vi "requireDataFromPort.vi"(3 "error in (no error)":errorcluster, 4 "Command":string, 5 "VISA resource name":refnum<visa-resource-name>="COM1" caption="端口号") -> (0 "error out":errorcluster, 1 "Data":string, 2 "VISA resource name 2":refnum<visa-resource-name>="COM1" caption="端口号")   [LabVIEW 2010]
panel:
  out "波形图表":dbl(graph)
  out "数值":dbl
  out "布尔":bool
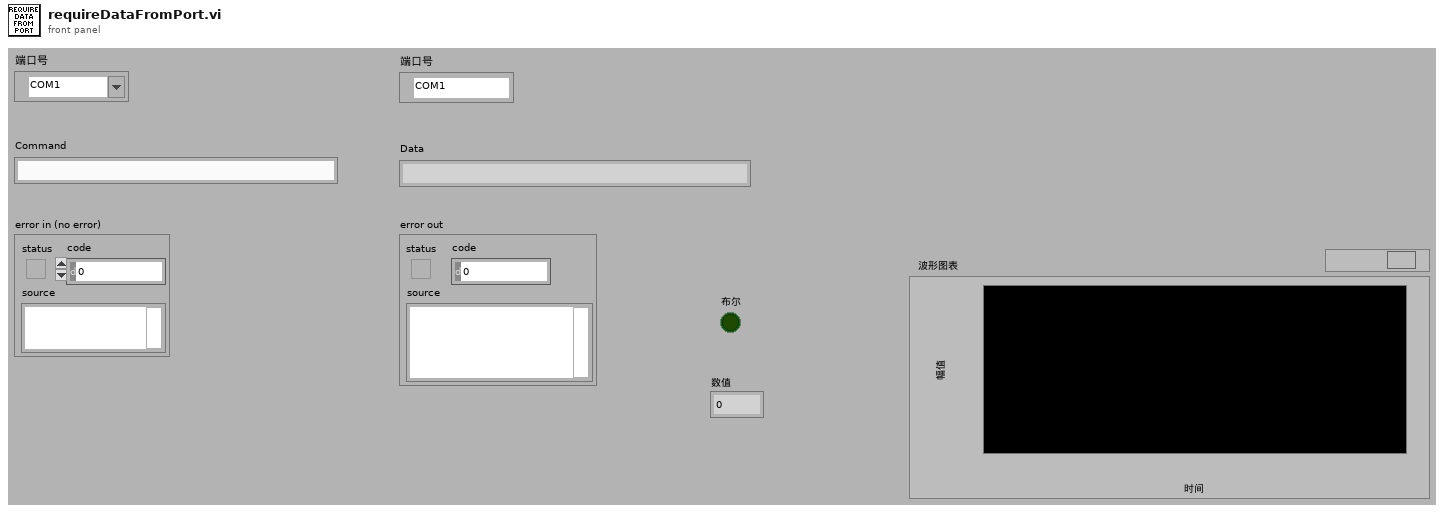
[diagram p1: front panel]
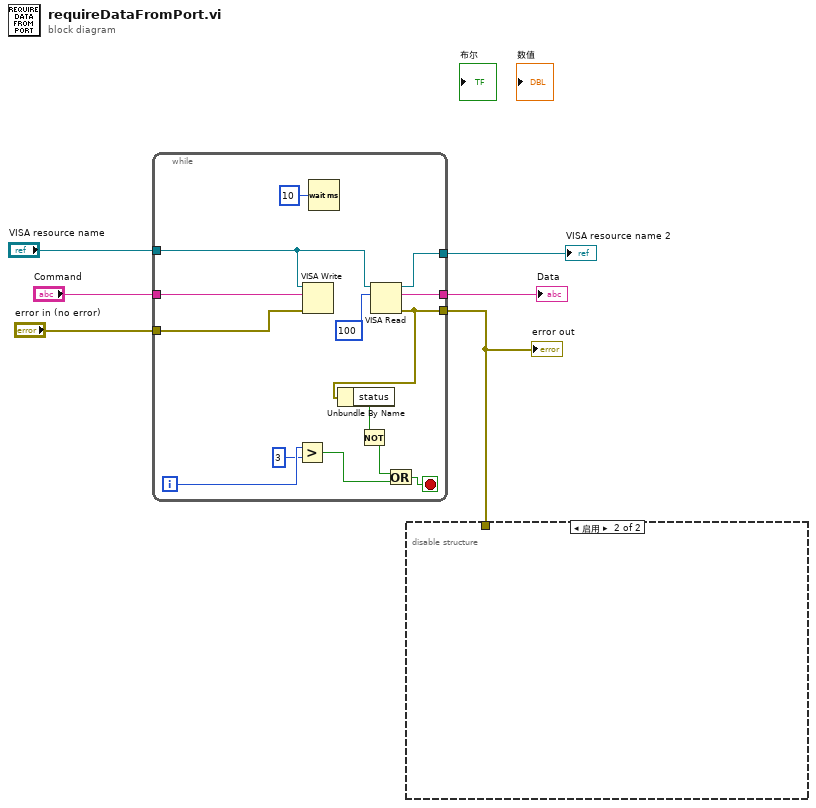
[diagram p0: block diagram]
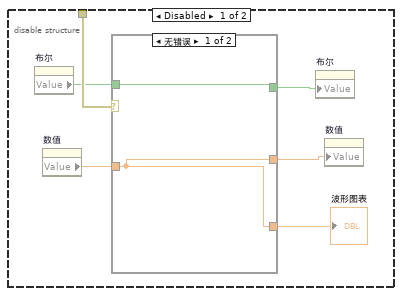
[diagram p2: hidden frame]
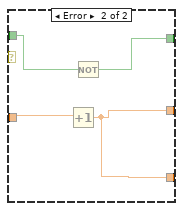
[diagram p3: hidden frame]
diagram:
  n1 = while {
    tunnel: "Command" -> [w19]
    tunnel: [w18] -> w5
    tunnel: [w17] -> w4
    tunnel: "error in (no error)" -> [w16]
    tunnel: "VISA resource name" -> [w15]
    tunnel: [w13] -> w1
    i -> [w12]
    stop <- w10 stop-if-true
    n2 = Greater?(x=w12, y=3) -> (0:w8:bool)
    n3 = VISA Write(VISA resource name=w15, write buffer=w19, error in (no error)=w16) -> ()  [unwired: 3 out]
    n4 = Wait (ms)(milliseconds to wait=u32 10 ("等待时间（毫秒）")) -> ()  [unwired: 1 out]
    n5 = VISA Read(VISA resource name=w15, byte count=u32 100 ("字节总数")) -> (VISA resource name out=w17:refnum<visa-resource-name>, read buffer=w18:string, error out=w13:errorcluster)  [unwired: 1 in, 1 out]
    n6 = Unbundle By Name(w13) -> ("status"=w9:bool)
    n7 = Not(x=w9) -> (.not. x?=w7:bool)
    n8 = Or(x=w7, y=w8) -> (x .or. y?=w10:bool)
  }
  "Data" <- w5
  "VISA resource name 2" <- w4
  "error out" <- w1
  n9 = disable-structure shown="启用" {
    disable-tunnel: w1 -> [w26 _]
    frame Disabled {
      n10 = property on="布尔" class="Bool (严格)"() -> ("Value"=w24:bool)  [unwired: 2 in, 2 out]
      n11 = property on="数值" class="DigNum (严格)"() -> ("Value"=w25:dbl)  [unwired: 2 in, 2 out]
      n12 = case shown="无错误" w26 {
        tunnel: w25 -> [w27 w30]
        tunnel: w24 -> [w28 w32]
        tunnel: [w28 w31] -> w23
        tunnel: [w27 w29] -> w22
        tunnel: [w27 w29] -> w21
        frame No Error {
        }
        frame Error {
          n13 = Increment(x=w30) -> (x+1=w29:dbl)
          n14 = Not(x=w32) -> (.not. x?=w31:bool)
        }
      }
      "波形图表" <- w21
      n15 = property on="布尔" class="Bool (严格)"("Value"=w23) -> ()  [unwired: 2 in, 2 out]
      n16 = property on="数值" class="DigNum (严格)"("Value"=w22) -> ()  [unwired: 2 in, 2 out]
    }
    frame Enabled {
    }
  }
